vi "average calculation2015.vi"() -> ()   [LabVIEW 2018]
uses:
  <vilib>/Analysis/baseanly.llb/Mean (DBL).vi
  <vilib>/Utility/file.llb/Read Delimited Spreadsheet (DBL).vi
  <vilib>/Analysis/NI_AALBase.lvlib
panel:
  out "Prepared by \nthe project":string
  out "Average Calculation":dbl
  out "Data":dbl[][](array[numeric])
  in  "Measurement file \nwith extension Txt":path
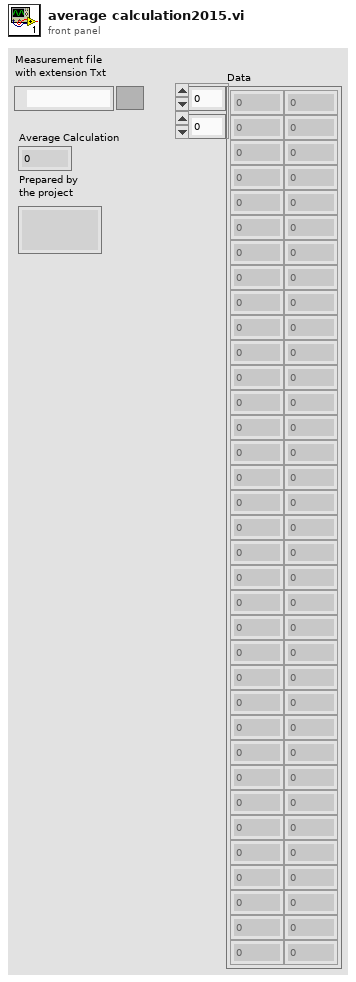
[diagram p1: front panel]
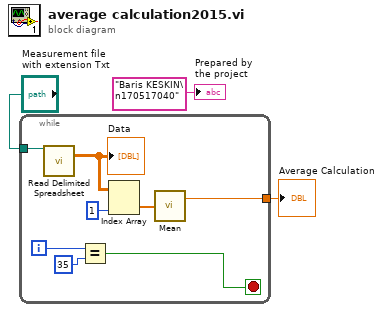
[diagram p0: block diagram]
diagram:
  n1 = while {
    tunnel: "Measurement file \nwith extension Txt" -> [w11]
    tunnel: [w7] -> w2
    i -> [w6]
    stop <- w4 stop-if-true
    n2 = call-poly <vilib>:"Read Delimited Spreadsheet.vi"("file path (dialog if empty)"=w11) -> ("all rows"=w9:dbl[][])  [unwired: 9 in, 5 out]
    "Data" <- w9
    n3 = Equal?(x=w6, y=35) -> (x = y?=w4:bool)
    n4 = Index Array(array=w9, index (col)=1 ("disabled index (col)")) -> (element=w8:dbl[])  [unwired: 1 in]
    n5 = call-poly <vilib>:"Mean.vi"("X"=w8) -> ("mean"=w7:dbl)  [unwired: 1 out]
  }
  "Average Calculation" <- w2
  "Prepared by \nthe project" <- "Baris KESKIN\n170517040"
